vi "New GUID.vi"() -> (3 "ToString":string)   [LabVIEW 2023, in "Redis Client Examples.lvlib"]
uses:
  Redis Client Examples.lvlib
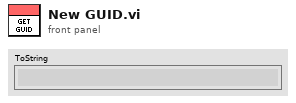
[diagram p1: front panel]
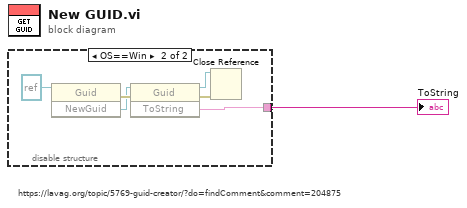
[diagram p0: block diagram]
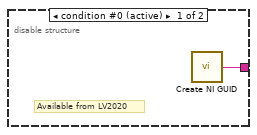
[diagram p2: hidden frame]
diagram:
  # "https://lavag.org/topic/5769-guid-creator/?do=findComment&comment=204875"
  n1 = disable-structure shown="OS==Win" {
    disable-tunnel: [w2 w4] -> w1
    frame condition #0 (active) {
      # "Available from LV2020"
      n2 = call <vilib>:"Create NI GUID.vi"() -> ("NI GUID"=w2:string)
    }
    frame condition #1 {
      n3 = invoke class="Guid" method="NewGuid"(reference=refnum<k24> refnum) -> (error out=w5:errorcluster, "NewGuid"=w3:refnum<k24>)  [unwired: 2 in, 1 out]
      n4 = invoke class="Guid" method="ToString"(reference=w3, error in=w5) -> (reference out=w7:refnum<k24>, error out=w6:errorcluster, "ToString"=w4:string)  [unwired: 1 in]
      n5 = Close Reference(reference=w7, error in (no error)=w6) -> ()  [unwired: 1 out]
    }
  }
  "ToString" <- w1
